vi "Configure Sampling points.vi"(8 "error in (no error)":errorcluster, 10 "Sampling points":i32=1001, 11 "VISA resource name":refnum<visa-resource-name>) -> (0 "error out":errorcluster, 3 "VISA resource name out":refnum<visa-resource-name>)   [LabVIEW 2021, in "Ceyear.lvlib"]
doc: "Configures the frequency range defining its start frequency and its stop frequency. If the start frequency is equal to the stop frequency, then the spectrum analyzer operates in the time-domain mode. Otherwise, the spectrum analyzer operates in frequency-domain mode."
uses:
  <instrlib>/Ceyear/Ceyear.lvlib
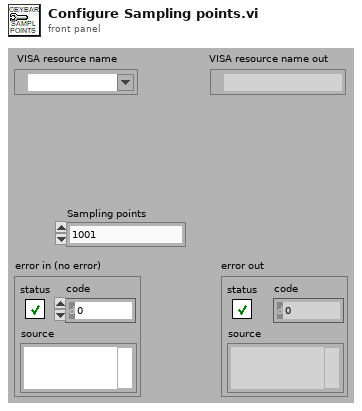
[diagram p1: front panel]
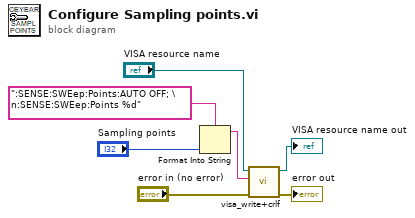
[diagram p0: block diagram]
diagram:
  n1 = Format Into String(format string=":SENSE:SWEep:Points:AUTO OFF; \n:SENSE:SWEep:Points %d", "Sampling points") -> (resulting string=w4:string)  [unwired: 2 in, 1 out]
  n2 = call <instrlib>:"visa_write+crlf.vi"("error in (no error)"="error in (no error)", "Strings (empty)"=w4, "VISA resource name"="VISA resource name") -> ("error out"=→"error out":errorcluster, "VISA resource name out"=→"VISA resource name out":refnum<visa-resource-name>)  [unwired: 7 in]
